vi "Car-matrix-poc.vi"() -> ()   [LabVIEW 2026]
uses:
  <vilib>/Utility/error.llb/Trim Whitespace One-Sided.vi
  CTI-Grove/Examples/Sourcecode/cti-drivers-lv-visa-simple/Examples/Driver/CTIPicoVISA.lvlib
panel:
  out "error out":errorcluster
  out "Identity":T1
  in  "VISA resource name in":refnum<visa-resource-name>
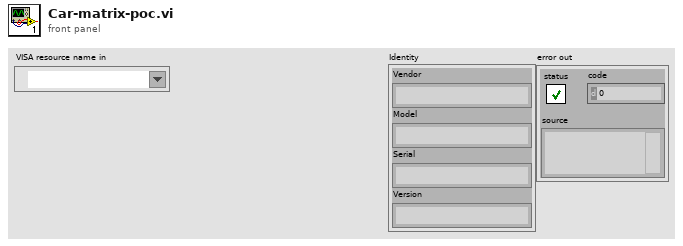
[diagram p1: front panel]
types:
  T1 = cluster{"Vendor":string, "Model":string, "Serial":string, "Version":string}
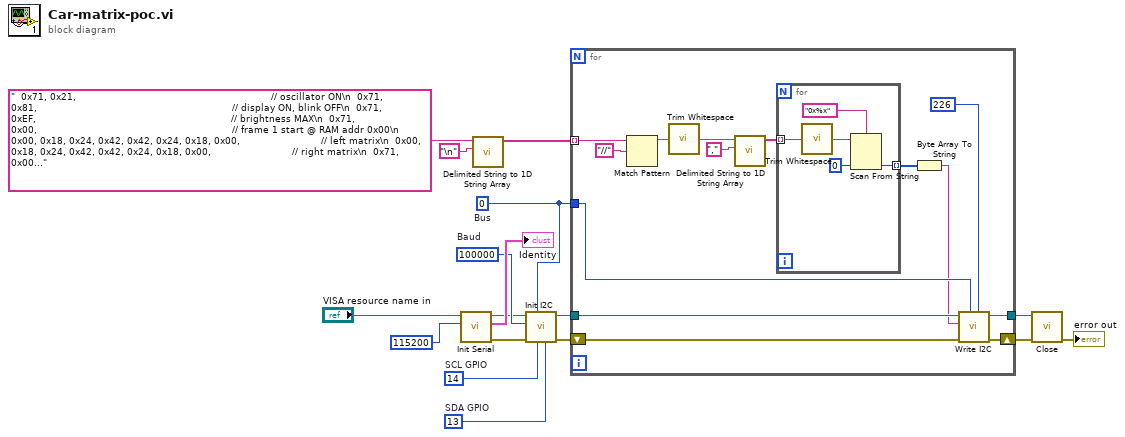
[diagram p0: block diagram]
diagram:
  w4 = u8 0  # Bus
  w10 = 13  # SDA GPIO
  w9 = 14  # SCL GPIO
  w8 = u32 100000  # Baud
  n1 = call "Init Serial.vi"("Baud (115200)"=u32 115200, "VISA resource name in"="VISA resource name in") -> ("error out"=w6:errorcluster, "Identity"=→"Identity":T1, "VISA resource name Out"=w7:refnum<visa-resource-name>)  [unwired: 7 in]
  n2 = call <vilib>:"Delimited String to 1D String Array.vi"("delimiter"="\n", "delimited string"="  0x71, 0x21,                                                                 // oscillator ON\n  0x71, 0x81,                                                                 // display ON, blink OFF\n  0x71, 0xEF,                                                                 // brightness MAX\n  0x71, 0x00,                                                                 // frame 1 start @ RAM addr 0x00\n  0x00, 0x18, 0x24, 0x42, 0x42, 0x24, 0x18, 0x00,                           // left matrix\n  0x00, 0x18, 0x24, 0x42, 0x42, 0x24, 0x18, 0x00,                           // right matrix\n  0x71, 0x00,                                                                 // frame 2 start @ RAM addr 0x00\n  0x00, 0x18, 0x24, 0x5A, 0x5A, 0x24, 0x18, 0x00,                           // left matrix\n  0x00, 0x18, 0x24, 0x5A, 0x5A, 0x24, 0x18, 0x00                            // right matrix") -> ("string array"=w5:string[])  [unwired: 9 in]
  n3 = call "Init I2C.vi"("SDA GPIO"=w10, "SCL GPIO"=w9, "Bus"=w4, "error in (no error)"=w6, "Baud"=w8, "VISA resource name in"=w7) -> ("error out"=w3:errorcluster, "VISA resource name"=w2:refnum<visa-resource-name>)  [unwired: 4 in]
  n4 = for {
    tunnel: [w22] -> w11
    tunnel: w5 -> [w31] mode=indexing
    tunnel: w4 -> [w25]
    tunnel: w2 -> [w23]
    shift-right: [w21] -> w1
    shift-left: w3 -> [w24]
    n5 = Match Pattern(string=w31, regular expression="//") -> (before substring=w29:string)  [unwired: 1 in, 3 out]
    n6 = call <vilib>:"Trim Whitespace.vi"("string"=w29) -> ("trimmed string"=w28:string)  [unwired: 1 in]
    n7 = call <vilib>:"Delimited String to 1D String Array.vi"("delimiter"=",", "delimited string"=w28) -> ("string array"=w26:string[])  [unwired: 9 in]
    n8 = for {
      tunnel: w26 -> [w35] mode=indexing
      tunnel: [w34] -> w19 mode=indexing
      n9 = call <vilib>:"Trim Whitespace.vi"("string"=w35) -> ("trimmed string"=w33:string)  [unwired: 1 in]
      n10 = Scan From String(format string="0x%x", input string=w33, default 1=u8 0 ("default value 1")) -> (output 1=w34:u8)  [unwired: 2 in, 3 out]
    }
    n11 = Byte Array To String(unsigned byte array=w19) -> (string=w20:string)
    n12 = call "Write I2C.vi"("Address"=u8 226, "Bus"=w25, "error in (no error)"=w24, "Data"=w20, "VISA resource name in"=w23) -> ("error out"=w21:errorcluster, "VISA resource name"=w22:refnum<visa-resource-name>)  [unwired: 5 in]
  }
  n13 = call "Close.vi"("error in (no error)"=w1, "VISA resource name in"=w11) -> ("error out"=→"error out":errorcluster)  [unwired: 9 in]
